vi "Do.vi"(8 "error in (no error)":errorcluster, 10 "Actor in":refnum<class "Actor.lvclass">, 11 "New Panel Launched Msg":refnum<class "New Panel Launched Msg.lvclass">) -> (0 "error out":errorcluster, 2 "Actor out":refnum<class "Actor.lvclass">)   [LabVIEW 2020, in "Chat Window Model.lvlib" / "New Panel Launched Msg.lvclass"]
doc: "This VI delivers the message to the actor by calling the appropriate method(s) on the actor."
uses:
  New Panel Launched Msg.lvclass
  C:/Users/huipeng8/Desktop/Chat-Window-Tutorial-Series/Video 11 - Actor Sub-panels/Chat Window UI Controller/Chat Window UI Controller Messages/UI Panel Launched Msg/UI Panel Launched Msg.lvclass
  <vilib>/ActorFramework/Actor/Actor.lvclass
  Chat Window Model/Chat Window Model.lvclass
  C:/Program Files/National Instruments/LabVIEW 2020/vi.lib/ActorFramework/Actor/Actor.lvclass
  Chat Window UI Controller/Chat Window UI Controller Messages/UI Panel Launched Msg/UI Panel Launched Msg.lvclass/UI Panel Launched Msg.ctl
  Chat Window UI Controller/Chat Window UI Controller Messages/UI Panel Launched Msg/UI Panel Launched Msg.lvclass
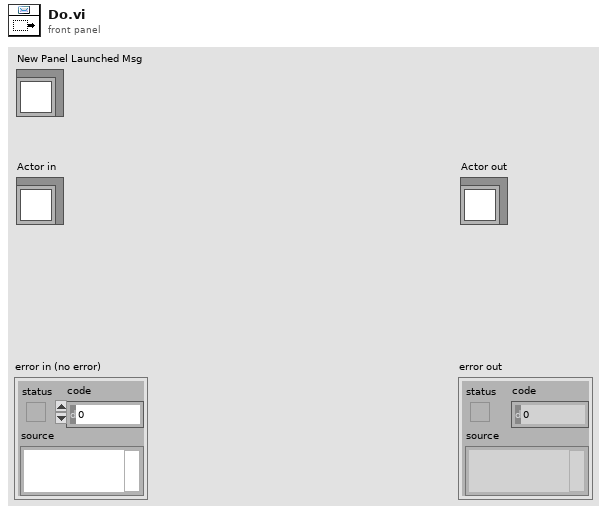
[diagram p1: front panel]
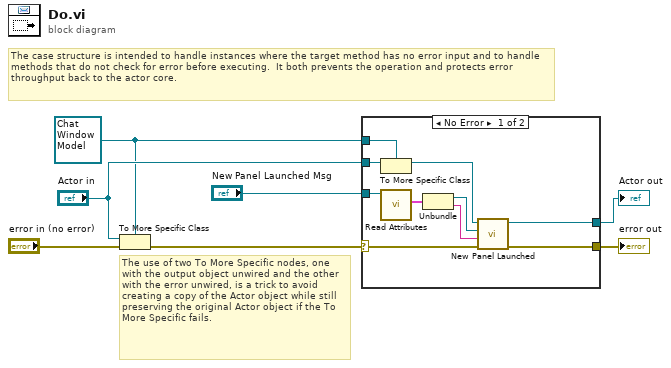
[diagram p0: block diagram]
diagram:
  w2 = refnum<class "Chat Window Model.lvclass"> refnum ("Actor in")
  # "The use of two To More Specific nodes, one with the output object unwired and the other with the error unwired, is a trick to avoid creating a copy of the Actor object while still preserving the original Actor object if the To More Specific fails."
  # "The case structure is intended to handle instances where the target method has no error input and to handle methods that do not check for error before executing.  It both prevents the operation and protects error throughput back to the actor core."
  n1 = To More Specific Class(target class=w2, reference="Actor in", error in="error in (no error)") -> (error out=w6:errorcluster)  [unwired: 1 out]
  n2 = case shown="No Error" w6 {
    selector: w6 -> [w15 w19]
    tunnel: [w17 w19] -> w5
    tunnel: [w16 w18] -> w4
    tunnel: "Actor in" -> [w14 w18]
    tunnel: w2 -> [w13 _]
    tunnel: "New Panel Launched Msg" -> [w10 _]
    frame No Error {
      n3 = To More Specific Class(target class=w13, reference=w14) -> (specific class reference=w12:refnum<class "Chat Window Model.lvclass">)  [unwired: 1 in, 1 out]
      n4 = call "Read Attributes.vi"("UI Panel Launched Msg"=w10) -> ("Payload"=w11:cluster{"VI Refnum":refnum<vi>, "Name":string})  [unwired: 10 in]
      n5 = Unbundle(w11) -> ("VI Refnum"=w9:refnum<vi>, "Name"=w8:string)
      n6 = call "New Panel Launched.vi"("error in (no error)"=w15, "Name"=w8, "VI Refnum"=w9, "Chat Window Model in"=w12) -> ("error out"=w17:errorcluster, "Chat Window Model out"=w16:refnum<class "Chat Window Model.lvclass">)  [unwired: 6 in]
    }
    frame Error {
      # "If type check fails, pass the original object out again."
    }
  }
  "error out" <- w5
  "Actor out" <- w4
